vi "Get_VI_Header_Info.vi"(0 "reference":refnum<vi>, 1 "error in (no error)":errorcluster) -> (2 "reference 2":refnum<vi>, 3 "Header info":T1={"page headers (unchanged)"=0, "page header content options"={"Include VI Name"=TRUE, "Include VI Path"=TRUE, "Include Last Modification Date"=TRUE, "Include Date Printed"=TRUE, "Include Page Number"=TRUE, "Include VI Icon"=TRUE}} {"page headers (unchanged)" items=["Unchanged", "Include page headers", "Do not include page headers"]}, 4 "error out":errorcluster)   [LabVIEW 2017, in "NI_ReportGenerationCore.lvlib"]
uses:
  <vilib>/Utility/NIReport.llb/NI_ReportGenerationCore.lvlib
  <vilib>/printing/EasyPrintingControls.llb/page_header_options.ctl
  <vilib>/printing/EasyPrintingControls.llb/page_headers.ctl
  <vilib>/printing/EasyPrintingControls.llb/page_header_content_options.ctl
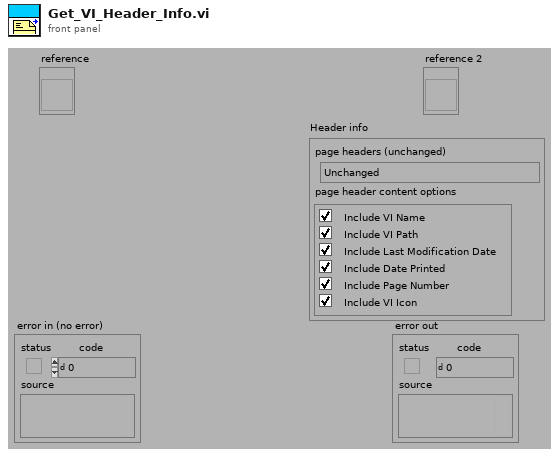
[diagram p1: front panel]
types:
  T1 = typedef "NI_ReportGenerationCore.lvlib/page_header_options.ctl" = cluster{"page headers (unchanged)":T2, "page header content options":T3}
  T2 = typedef "NI_ReportGenerationCore.lvlib/page_headers.ctl" = u16
  T3 = typedef "NI_ReportGenerationCore.lvlib/page_header_content_options.ctl" = cluster{"Include VI Name":bool, "Include VI Path":bool, "Include Last Modification Date":bool, "Include Date Printed":bool, "Include Page Number":bool, "Include VI Icon":bool}
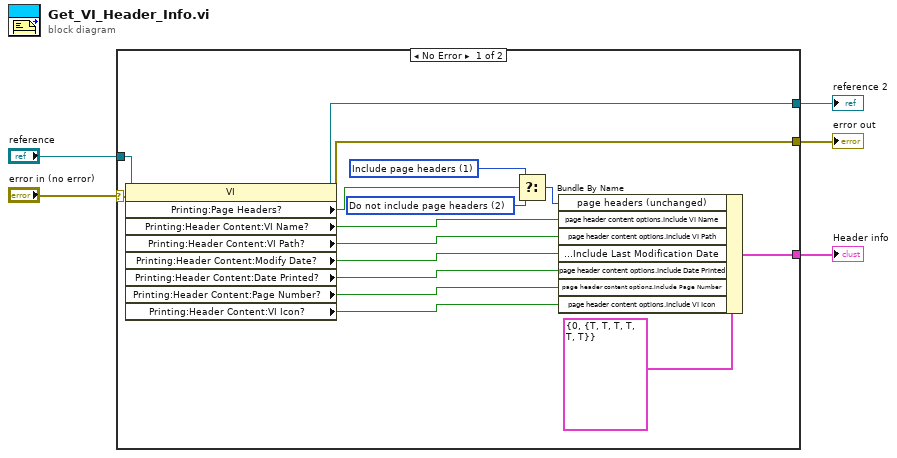
[diagram p0: block diagram]
diagram:
  n1 = case shown="No Error" "error in (no error)" {
    selector: "error in (no error)" -> [w19 w22]
    tunnel: "reference" -> [w6 w23]
    tunnel: [w21 w23] -> w4
    tunnel: [w20 w22] -> w3
    tunnel: [w9 _] -> w1
    frame No Error {
      w7 = T2 2 items=["Unchanged", "Include page headers", "Do not include page headers"] ("page headers (unchanged)")
      w8 = T2 1 items=["Unchanged", "Include page headers", "Do not include page headers"] ("page headers (unchanged)")
      n2 = property class="VI"(reference=w6, error in=w19) -> (reference out=w21:refnum<vi>, error out=w20:errorcluster, "Printing:Page Headers?"=w17:bool, "Printing:Header Content:VI Name?"=w15:bool, "Printing:Header Content:VI Path?"=w14:bool, "Printing:Header Content:Modify Date?"=w13:bool, "Printing:Header Content:Date Printed?"=w12:bool, "Printing:Header Content:Page Number?"=w11:bool, "Printing:Header Content:VI Icon?"=w10:bool)
      n3 = Select(t=w8, s=w17, f=w7) -> (s? t:f=w16:T2)
      n4 = Bundle By Name(cluster=T1 {"page headers (unchanged)"=0, "page header content options"={"Include VI Name"=TRUE, "Include VI Path"=TRUE, "Include Last Modification Date"=TRUE, "Include Date Printed"=TRUE, "Include Page Number"=TRUE, "Include VI Icon"=TRUE}} ("page header options"), "page headers (unchanged)"=w16, "page header content options.Include VI Name"=w15, "page header content options.Include VI Path"=w14, "page header content options.Include Last Modification Date"=w13, "page header content options.Include Date Printed"=w12, "page header content options.Include Page Number"=w11, "page header content options.Include VI Icon"=w10) -> (w9:T1)
    }
    frame Error {
    }
  }
  "reference 2" <- w4
  "error out" <- w3
  "Header info" <- w1
